vi "coagBuffer.vi"(6 "command":T1=enum."read recent", 7 "all data in":cluster{"time":timestamp[], "all coag in":dbl[]}, 8 "error in (no error)":errorcluster, 9 "Time Stamp":timestamp, 10 "max array size":u16=5000 min=1, 11 "Coag dose":dbl) -> (0 "error out":errorcluster, 2 "all data out":cluster{"time":timestamp[], "all coag in":dbl[]}, 3 "recent coag":dbl)   [LabVIEW 2015]
uses:
  coagbuffer.ctl
panel:
  out "recent time":timestamp
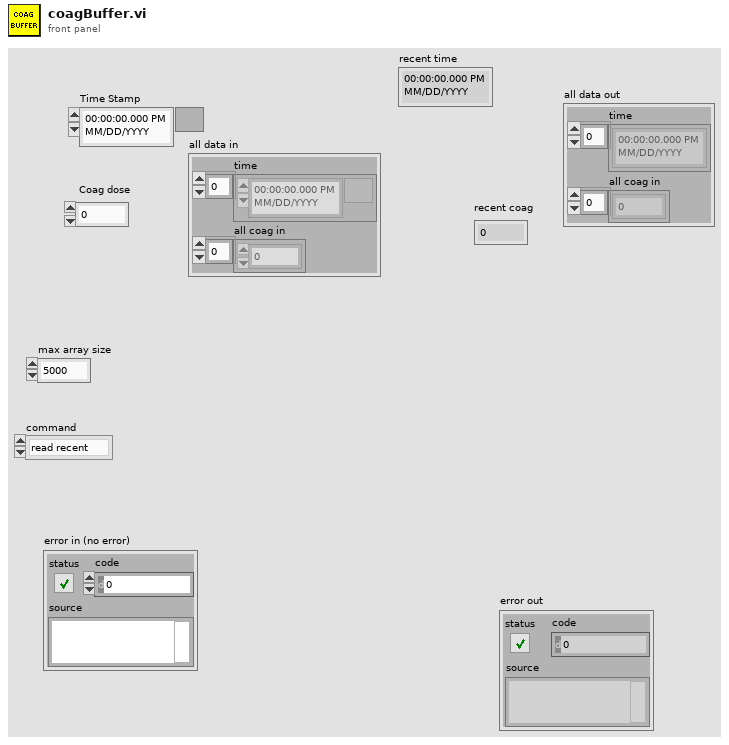
[diagram p1: front panel]
types:
  T1 = typedef "coagbuffer.ctl" = enum16{"set buffer size", "write", "refill buffer", "read recent", "read all", "clear", "overwrite"}
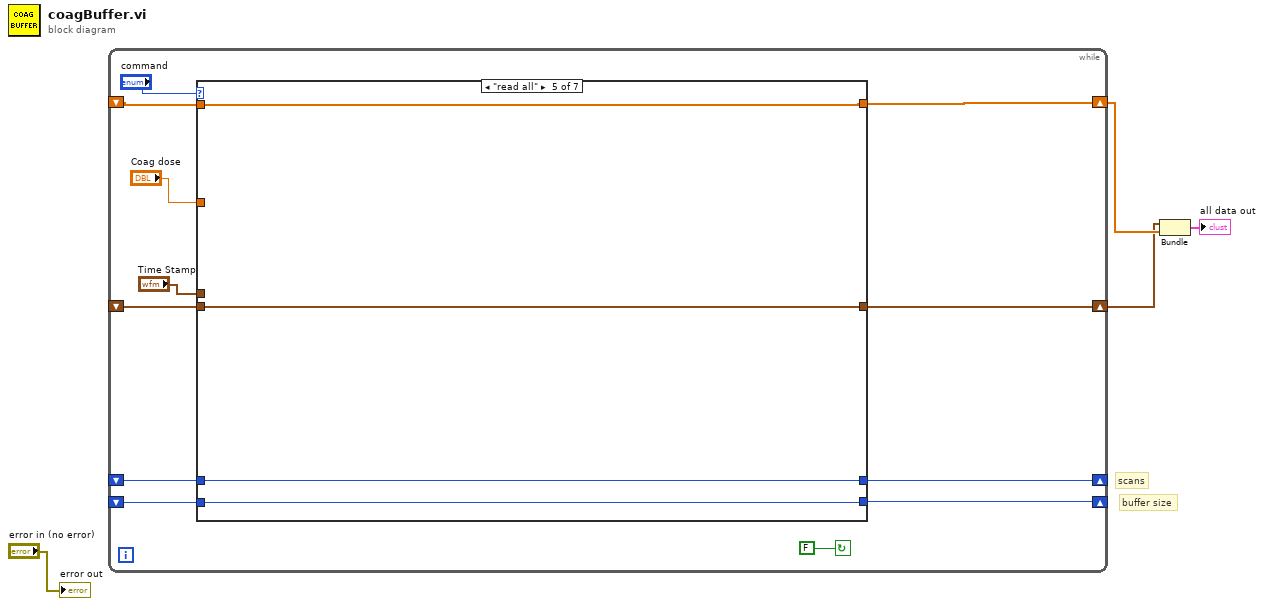
[diagram p0: block diagram]
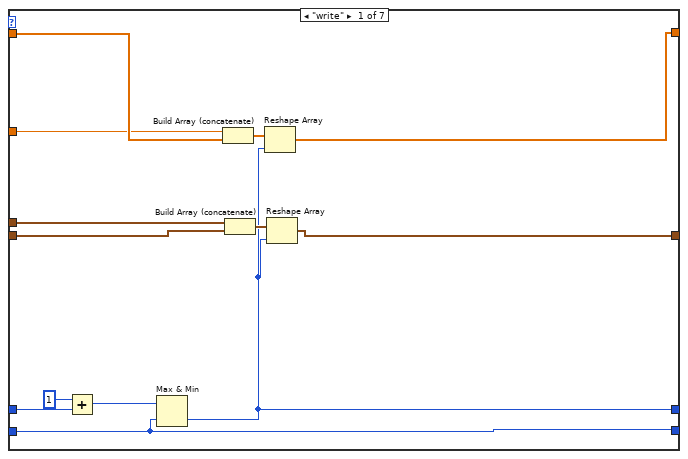
[diagram p2: hidden frame]
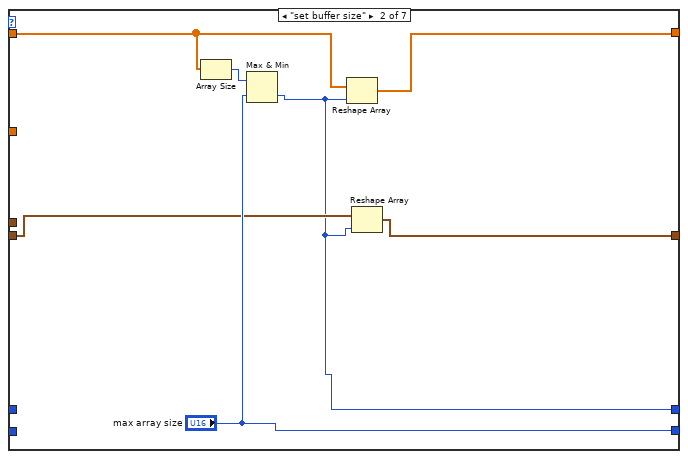
[diagram p3: hidden frame]
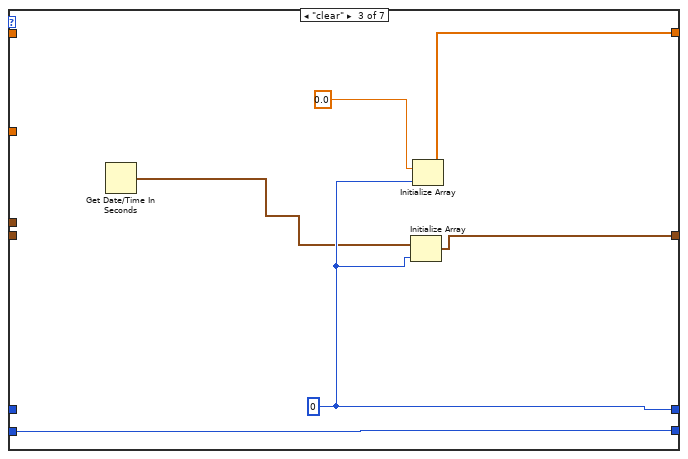
[diagram p4: hidden frame]
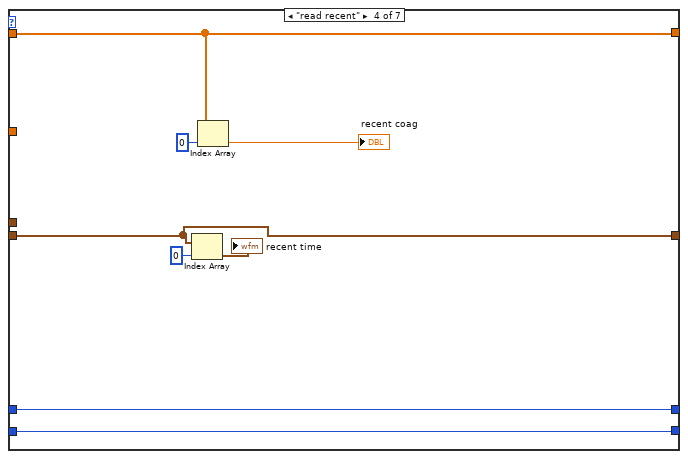
[diagram p5: hidden frame]
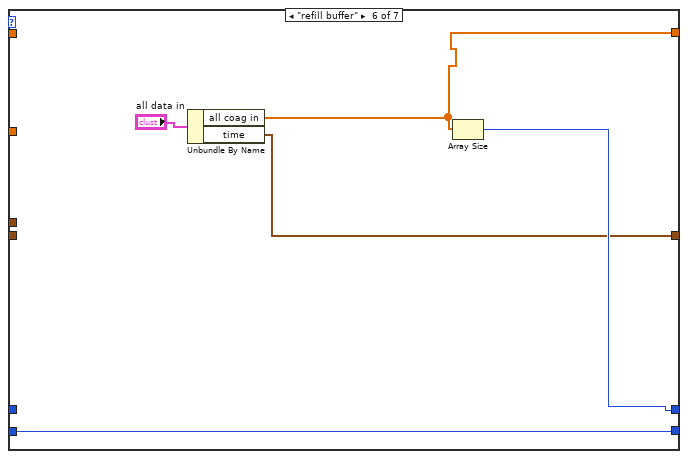
[diagram p6: hidden frame]
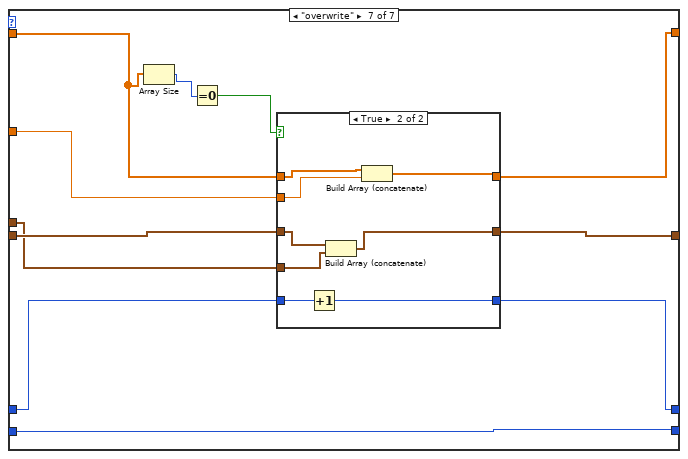
[diagram p7: hidden frame]
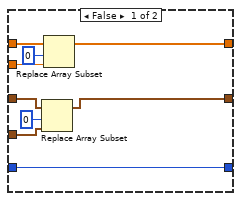
[diagram p8: hidden frame]
diagram:
  # "buffer size"
  # "scans"
  n1 = while {
    shift-right: [w15] -> w2
    shift-left: _ -> [w14]
    shift-right: [w13] -> _
    shift-left: _ -> [w12]
    shift-right: [w9] -> _
    shift-left: _ -> [w10]
    shift-right: [w7] -> w1
    shift-left: _ -> [w6]
    stop <- FALSE continue-if-true
    n2 = case shown="\"read all\"" "command" {
      tunnel: [w26 w36 w42 w50 w51 w56 w68] -> w15
      tunnel: w14 -> [w28 w35 _ w50 w51 _ w64]
      tunnel: [w23 "max array size" w41 w48 w54 w59 w70] -> w13
      tunnel: w12 -> [w23 _ w41 w48 w54 w59 w70]
      tunnel: w10 -> [w27 _ _ w47 w53 _ w61]
      tunnel: [w20 w31 w39 w47 w53 w58 w60] -> w9
      tunnel: "Coag dose" -> [w22 _ _ _ _ _ w69]
      tunnel: [w19 w30 w38 w43 w52 w55 w65] -> w7
      tunnel: w6 -> [w18 w32 _ w43 w52 _ w67]
      tunnel: "Time Stamp" -> [w17 _ _ _ _ _ w66]
      frame "write" {
        n3 = Add(x=1, y=w27) -> (x+y=w24:i32)
        n4 = Max & Min(x=w24, y=w23) -> (min(x,y)=w20:i32)  [unwired: 1 out]
        n5 = Build Array (concatenate)(w22, w28) -> (w25:dbl[])
        n6 = Build Array (concatenate)(w17, w18) -> (w21:timestamp[])
        n7 = Reshape Array(w25, w20) -> (w26:dbl[])
        n8 = Reshape Array(w21, w20) -> (w19:timestamp[])
      }
      frame "set buffer size" {
        n9 = Array Size(array=w35) -> (size(s)=w34:i32)
        n10 = Max & Min(x=w34, y="max array size") -> (min(x,y)=w31:i32)  [unwired: 1 out]
        n11 = Reshape Array(w35, w31) -> (w36:dbl[])
        n12 = Reshape Array(w32, w31) -> (w30:timestamp[])
      }
      frame "clear" {
        w39 = 0
        n13 = Get Date/Time In Seconds() -> (seconds since 1Jan1904=w37:timestamp)
        n14 = Initialize Array(w37, w39) -> (w38:timestamp[])
        n15 = Initialize Array(0.0, w39) -> (w42:dbl[])
      }
      frame "read recent" {
        n16 = Index Array(array=w43, index=0) -> (element=→"recent time":timestamp)
        n17 = Index Array(array=w50, index=0) -> (element=→"recent coag":dbl)
      }
      frame "read all" {
      }
      frame "refill buffer" {
        n18 = Unbundle By Name("all data in") -> ("all coag in"=w56:dbl[], "time"=w55:timestamp[])
        n19 = Array Size(array=w56) -> (size(s)=w58:i32)
      }
      frame "overwrite" {
        n20 = Array Size(array=w64) -> (size(s)=w63:i32)
        n21 = Equal To 0?(x=w63) -> (x = 0?=w62:bool)
        n22 = case shown="True" w62 {
          tunnel: w69 -> [w79 w87]
          tunnel: [w78 w85] -> w68
          tunnel: w67 -> [w75 w84]
          tunnel: w66 -> [w74 w83]
          tunnel: [w73 w82] -> w65
          tunnel: w64 -> [w72 w86]
          tunnel: w61 -> [w71 w81]
          tunnel: [w71 w80] -> w60
          frame False {
            n23 = Replace Array Subset(array=w75, new element=w74, index=0) -> (w73:timestamp[])
            n24 = Replace Array Subset(array=w72, new element=w79, index=0) -> (w78:dbl[])
          }
          frame True {
            n25 = Increment(x=w81) -> (x+1=w80:i32)
            n26 = Build Array (concatenate)(w84, w83) -> (w82:timestamp[])
            n27 = Build Array (concatenate)(w86, w87) -> (w85:dbl[])
          }
        }
      }
    }
  }
  n28 = Bundle("time"=w1, "all coag in"=w2) -> (→"all data out":cluster{"time":timestamp[], "all coag in":dbl[]})  [unwired: 1 in]
  "error out" <- "error in (no error)"
